vi "Check If Parent Missile.vi"(9 "GB Components in":refnum<class "Game Board Component.lvclass">[](array[class]), 11 "Missile in":refnum<class "Missile.lvclass">) -> (2 "Not parent missile?":bool)   [LabVIEW 2021, in "Missile.lvclass"]
doc: "MIT Licence\nCopyright (c) 2024 David Grollier"
uses:
  Missile.lvclass
  Game Board Component.lvclass
  Game Board Component.lvclass/Game Board Component.ctl
  Missile.lvclass/Missile.ctl
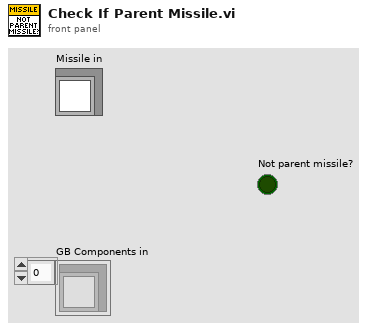
[diagram p1: front panel]
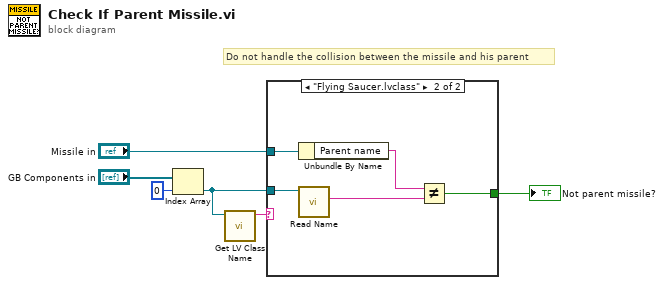
[diagram p0: block diagram]
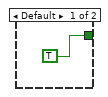
[diagram p2: hidden frame]
diagram:
  # "Do not handle the collision between the missile and his parent"
  n1 = Index Array(array="GB Components in", index=0) -> (element=w2:refnum<class "Game Board Component.lvclass">)
  n2 = call <vilib>:"Get LV Class Name.vi"("object"=w2) -> ("class name"=w4:string)  [unwired: 9 in, 1 out]
  n3 = case shown="\"Flying Saucer.lvclass\"" w4 {
    tunnel: [TRUE w8] -> w3
    tunnel: w2 -> [_ w12]
    tunnel: "Missile in" -> [_ w11]
    frame Default {
    }
    frame "Flying Saucer.lvclass" {
      n4 = Unbundle By Name(w11) -> ("Parent name"=w10:string)
      n5 = call "Read Name.vi"("Game Board Component in"=w12) -> ("Name"=w9:string)  [unwired: 10 in]
      n6 = Not Equal?(x=w10, y=w9) -> (x != y?=w8:bool)
    }
  }
  "Not parent missile?" <- w3
